vi "Autonomous Mode.vi"(0 "Drive Motors":string="RobotDrive", 5 "B.Pick up":string="My Motor RefNum", 7 "A.Pick up":string="My Solenoid RefNum", 9 "Shooter":string="My Motor RefNum", 11 "Inverted Shooter":string="My Motor RefNum") -> ()   [LabVIEW 2013]
uses:
  <vilib>/Rock Robotics/WPI/Solenoid/WPI_SolenoidValue.ctl
  Auton Mode Determiner.vi
  <vilib>/Rock Robotics/WPI/Compressor/WPI_CompressorGetSetRefNum.vi
  <vilib>/Rock Robotics/WPI/RobotDrive/WPI_RobotDriveGetSetRefNum.vi
  Ultrasonic Sensor.vi
  <vilib>/Rock Robotics/WPI/RobotDrive/WPI_RobotDriveArcadeDrive_Standard(NoSaturation).vi
  <vilib>/Rock Robotics/WPI/Solenoid/Deprecated/WPI_SolenoidGetBool.vi
  <vilib>/Rock Robotics/WPI/Solenoid/WPI_SolenoidSetEnum.vi
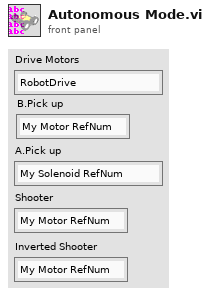
[diagram p1: front panel]
types:
  T1 = typedef "WPI_CompressorDevRef.ctl" = cluster{"DevStatus":errorcluster, "DigitalInputDevRef":T2, "RelayDevRef":T5}
  T2 = typedef "WPI_DigitalInputDevRef.ctl" = cluster{"DevStatus":errorcluster, "DIO Channel":T3, "Digital Module":T4}
  T3 = typedef "FPGA_DIOChannel.ctl" = enum8{"DIO 1", "DIO 2", "DIO 3", "DIO 4", "DIO 5", "DIO 6", "DIO 7", "DIO 8", "DIO 9", "DIO 10", "DIO 11", "DIO 12", "DIO 13", "DIO 14", "Invalid"}
  T4 = typedef "FPGA_TypedefDigitalModule.ctl" = enum16{"Digital Module 1", "Digital Module 2"}
  T5 = typedef "WPI_RelayDevRef.ctl" = cluster{"DevStatus":errorcluster, "Relay Channel":T6, "Digital Module":T4, "Relay Direction":T7}
  T6 = typedef "FPGA_DIORelayChannel.ctl" = enum8{"Relay 1", "Relay 2", "Relay 3", "Relay 4", "Relay 5", "Relay 6", "Relay 7", "Relay 8", "Invalid"}
  T7 = typedef "WPI_RelayDirection.ctl" = enum16{"Both directions", "Forward only", "Reverse only"}
  T8 = typedef "WPI_MotorControlDeviceRef.ctl" = cluster{"DeviceStatus":errorcluster, "Type":enum16{"PWM", "CAN"}, "PWM":cluster{"Digital Module":T4, "PWM Channel":T9, "DeadBand":T10}, "CAN":cluster{"Device Number":u8, "Control Mode":T11, "Semaphore":T12, "Max Vout":dbl}, "Invert":bool, "TransformRef":T13, "InvTransformRef":T13}
  T9 = typedef "FPGA_DIOPWMChannel.ctl" = enum8{"PWM 1", "PWM 2", "PWM 3", "PWM 4", "PWM 5", "PWM 6", "PWM 7", "PWM 8", "PWM 9", "PWM 10", "Invalid"}
  T10 = typedef "WPI_PWMDeadband.ctl" = cluster{"Name":string, "maxPositivePwm":i32, "minPositivePwm":i32, "centerPwm":i32, "maxNegativePwm":i32, "minNegativePwm":i32, "angularRange":u16}
  T11 = typedef "WPI_CANJaguar_ControlMode.ctl" = enum8{"Percent VBus", "Current", "Speed", "Position", "Voltage"}
  T12 = typedef "Semaphore RefNum" = refnum<k1>
  T13 = typedef "WPI_PWMTransform_ConPane.ctl" = refnum<vi>
  T14 = typedef "WPI_SolenoidDevRef.ctl" = cluster{"DevStatus":errorcluster, "Solenoid Module":T15, "Forward Solenoid Channel":T16, "Reverse Solenoid Channel":T16}
  T15 = typedef "FPGA_TypedefSolenoidModule.ctl" = enum16{"Solenoid Module 1", "Solenoid Module 2"}
  T16 = typedef "WPI_SolenoidChannel.ctl" = enum8{"Solenoid 1", "Solenoid 2", "Solenoid 3", "Solenoid 4", "Solenoid 5", "Solenoid 6", "Solenoid 7", "Solenoid 8", "Invalid"}
  T17 = typedef "WPI_RobotDriveDevRef.ctl" = cluster{"DevStatus":errorcluster, "Motors[]":T8[], "Square Inputs":bool, "Max Output":dbl, "Isochronous":bool}
  T18 = typedef "WPI_SolenoidValue.ctl" = enum16{"Off", "On", "Forward", "Reverse"}
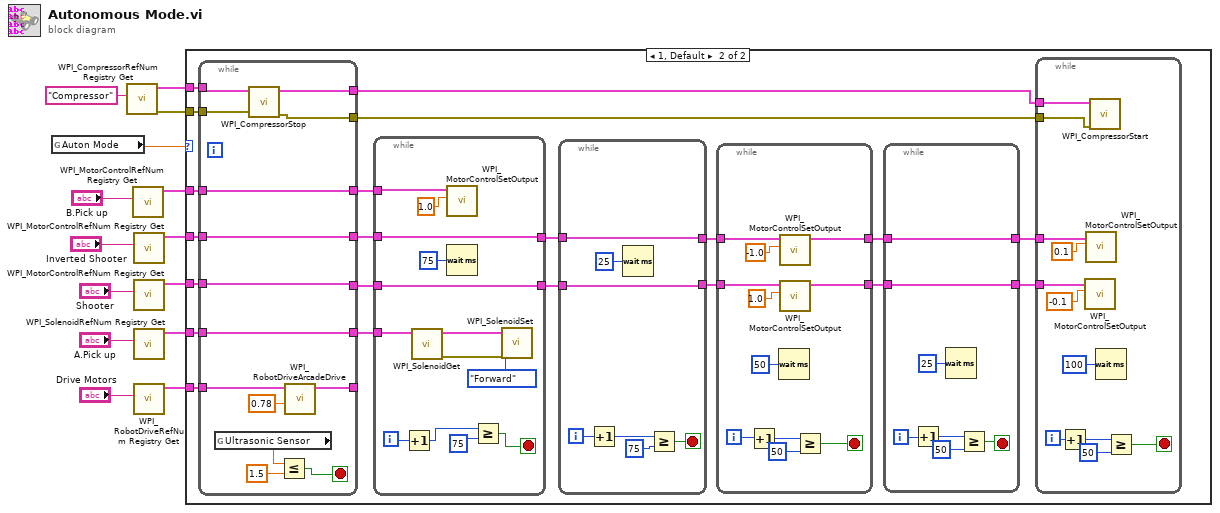
[diagram p0: block diagram]
diagram:
  n1 = global read "Auton Mode Determiner.vi" "Auton Mode"() -> (w4:dbl)
  n2 = call <vilib>:"WPI_CompressorRefNum Registry Get.vi"("refnum name"="Compressor") -> ("error out"=w2:errorcluster, "CompressorDevRef"=w3:T1)  [unwired: 9 in]
  n3 = call <vilib>:"WPI_MotorControlRefNum Registry Get.vi"("refnum name"="B.Pick up") -> ("MotorControlDevRef"=w5:T8)  [unwired: 9 in, 1 out]
  n4 = call <vilib>:"WPI_MotorControlRefNum Registry Get.vi"("refnum name"="Inverted Shooter") -> ("MotorControlDevRef"=w6:T8)  [unwired: 9 in, 1 out]
  n5 = call <vilib>:"WPI_MotorControlRefNum Registry Get.vi"("refnum name"="Shooter") -> ("MotorControlDevRef"=w7:T8)  [unwired: 9 in, 1 out]
  n6 = call <vilib>:"WPI_SolenoidRefNum Registry Get.vi"("refnum name"="A.Pick up") -> ("SolenoidDevRef"=w11:T14)  [unwired: 9 in, 1 out]
  n7 = call <vilib>:"WPI_RobotDriveRefNum Registry Get.vi"("refnum name"="Drive Motors") -> ("RobotDriveDevRef"=w14:T17)  [unwired: 9 in, 1 out]
  n8 = case shown="1, Default" w4 {
    tunnel: w14 -> [_ w35]
    tunnel: w11 -> [_ w34]
    tunnel: w7 -> [_ w33]
    tunnel: w6 -> [_ w32]
    tunnel: w5 -> [_ w31]
    tunnel: w3 -> [_ w18]
    tunnel: w2 -> [_ w17]
    frame 0 {
    }
    frame 1, Default {
      n9 = while {
        tunnel: [w98] -> _
        tunnel: w35 -> [w97]
        tunnel: w34 -> [w96]
        tunnel: [w96] -> w30
        tunnel: [w95] -> w27
        tunnel: w33 -> [w95]
        tunnel: [w94] -> w28
        tunnel: w32 -> [w94]
        tunnel: [w93] -> w29
        tunnel: w31 -> [w93]
        tunnel: w18 -> [w85]
        tunnel: w17 -> [w88]
        tunnel: [w87] -> w16
        tunnel: [w86] -> w15
        stop <- w90 stop-if-true
        n10 = global read "Ultrasonic Sensor.vi" "Ultrasonic Sensor"() -> (w92:dbl)
        n11 = call <vilib>:"WPI_CompressorStop.vi"("error in (no error)"=w88, "CompressorDevRef"=w85) -> ("error out"=w87:errorcluster, "CompressorDevRef"=w86:T1)  [unwired: 8 in]
        n12 = Less Or Equal?(x=w92, y=1.5) -> (x <= y?=w90:bool)
        n13 = call-poly <vilib>:"WPI_RobotDriveArcadeDrive.vi"("Y axis value"=0.78, "RobotDriveDevRef"=w97) -> ("RobotDriveDevRef"=w98:T17)  [unwired: 7 in, 2 out]
      }
      n14 = while {
        tunnel: w30 -> [w84]
        tunnel: w29 -> [w76]
        tunnel: w28 -> [w72]
        tunnel: w27 -> [w73]
        tunnel: [w73] -> w26
        tunnel: [w72] -> w25
        i -> [w83]
        stop <- w80 stop-if-true
        n15 = Increment(x=w83) -> (x+1=w82:i32)
        n16 = call-poly <vilib>:"WPI_SolenoidGet.vi"("SolenoidDevRef"=w84) -> ("error out"=w79:errorcluster, "SolenoidDevRef"=w78:T14)  [unwired: 8 in, 1 out]
        n17 = call <vilib>:"WPI_MotorControlSetOutput.vi"("Output"=1.0, "MotorControlDevRef"=w76) -> ()  [unwired: 7 in, 3 out]
        n18 = Wait (ms)(milliseconds to wait=u32 75) -> ()  [unwired: 1 out]
        n19 = Greater Or Equal?(x=w82, y=75) -> (x >= y?=w80:bool)
        n20 = call-poly <vilib>:"WPI_SolenoidSet.vi"("error in (no error)"=w79, "Value"=WPI_SolenoidValue."Forward", "SolenoidDevRef"=w78) -> ()  [unwired: 7 in, 2 out]
      }
      n21 = while {
        tunnel: [w67] -> w24
        tunnel: w26 -> [w67]
        tunnel: w25 -> [w66]
        tunnel: [w66] -> w23
        i -> [w68]
        stop <- w69 stop-if-true
        n22 = Increment(x=w68) -> (x+1=w70:i32)
        n23 = Wait (ms)(milliseconds to wait=u32 25) -> ()  [unwired: 1 out]
        n24 = Greater Or Equal?(x=w70, y=75) -> (x >= y?=w69:bool)
      }
      n25 = while {
        tunnel: w24 -> [w59]
        tunnel: w23 -> [w60]
        tunnel: [w56] -> w22
        tunnel: [w55] -> w21
        i -> [w64]
        stop <- w61 stop-if-true
        n26 = Increment(x=w64) -> (x+1=w63:i32)
        n27 = Wait (ms)(milliseconds to wait=u32 50) -> ()  [unwired: 1 out]
        n28 = call <vilib>:"WPI_MotorControlSetOutput.vi"("Output"=-1.0, "MotorControlDevRef"=w60) -> ("MotorControlDevRef"=w55:T8)  [unwired: 7 in, 2 out]
        n29 = call <vilib>:"WPI_MotorControlSetOutput.vi"("Output"=1.0, "MotorControlDevRef"=w59) -> ("MotorControlDevRef"=w56:T8)  [unwired: 7 in, 2 out]
        n30 = Greater Or Equal?(x=w63, y=50) -> (x >= y?=w61:bool)
      }
      n31 = while {
        tunnel: w22 -> [w47]
        tunnel: w21 -> [w48]
        tunnel: [w48] -> w20
        tunnel: [w47] -> w19
        i -> [w51]
        stop <- w50 stop-if-true
        n32 = Increment(x=w51) -> (x+1=w53:i32)
        n33 = Wait (ms)(milliseconds to wait=u32 25) -> ()  [unwired: 1 out]
        n34 = Greater Or Equal?(x=w53, y=50) -> (x >= y?=w50:bool)
      }
      n35 = while {
        tunnel: w20 -> [w46]
        tunnel: w19 -> [w45]
        tunnel: w16 -> [w37]
        tunnel: w15 -> [w36]
        i -> [w42]
        stop <- w41 stop-if-true
        n36 = Increment(x=w42) -> (x+1=w43:i32)
        n37 = call <vilib>:"WPI_MotorControlSetOutput.vi"("Output"=-0.1, "MotorControlDevRef"=w45) -> ()  [unwired: 7 in, 3 out]
        n38 = call <vilib>:"WPI_MotorControlSetOutput.vi"("Output"=0.1, "MotorControlDevRef"=w46) -> ()  [unwired: 7 in, 3 out]
        n39 = call <vilib>:"WPI_CompressorStart.vi"("error in (no error)"=w37, "CompressorDevRef"=w36) -> ()  [unwired: 8 in, 2 out]
        n40 = Wait (ms)(milliseconds to wait=u32 100) -> ()  [unwired: 1 out]
        n41 = Greater Or Equal?(x=w43, y=50) -> (x >= y?=w41:bool)
      }
    }
  }
